vi "cargoLoop.vi"() -> ()   [LabVIEW 2018]
uses:
  <vilib>/Platform/TimedLoop/XDataNode/timing_clust.ctl
  <vilib>/Platform/TimedLoop/XDataNode/nitl_modes.ctl
  <vilib>/Platform/TimedLoop/XDataNode/wakeup.ctl
  <vilib>/Rock Robotics/WPI/Solenoid/WPI_SolenoidValue.ctl
  cargoNotifier.ctl
  cargoEnum.ctl
  <userlib>/836-Library/System/TDMS_V2/Support/TDMS_DevRef.ctl
  <userlib>/836-Library/System/TDMS_V2/Support/Logging_Settings.ctl
  <userlib>/836-Library/System/TDMS_V2/Support/Group_FIFO_Config.ctl
  <userlib>/836-Library/System/TDMS_V2/Support/Channel_FIFO_Config.ctl
  <vilib>/Rock Robotics/WPI/Solenoid/WPI_SolenoidSetEnum.vi
  <vilib>/platform/TimedLoop/XDataNode/XDataNode.xnode
  <vilib>/Platform/TimedLoop/XDataNode/XDNodeRunTimeDep.lvlib
panel:
  in  "Cargo_Shoot_Time Left":dbl=0.16
  in  "Shoot Time Low Rocket":dbl=1.0
  in  "Cargo_Shoot_Time Right":dbl=0.04
  in  "Rocket_High_Shoot_Time":dbl=1.0
  in  "Reset":bool
  out "Data":cluster{i16, i16}(graph)={1, 0}
  out "Right_Out":bool
  out "Left_Out":bool
  out "Shoot_Right?":bool
  out "Shoot_Left?":bool
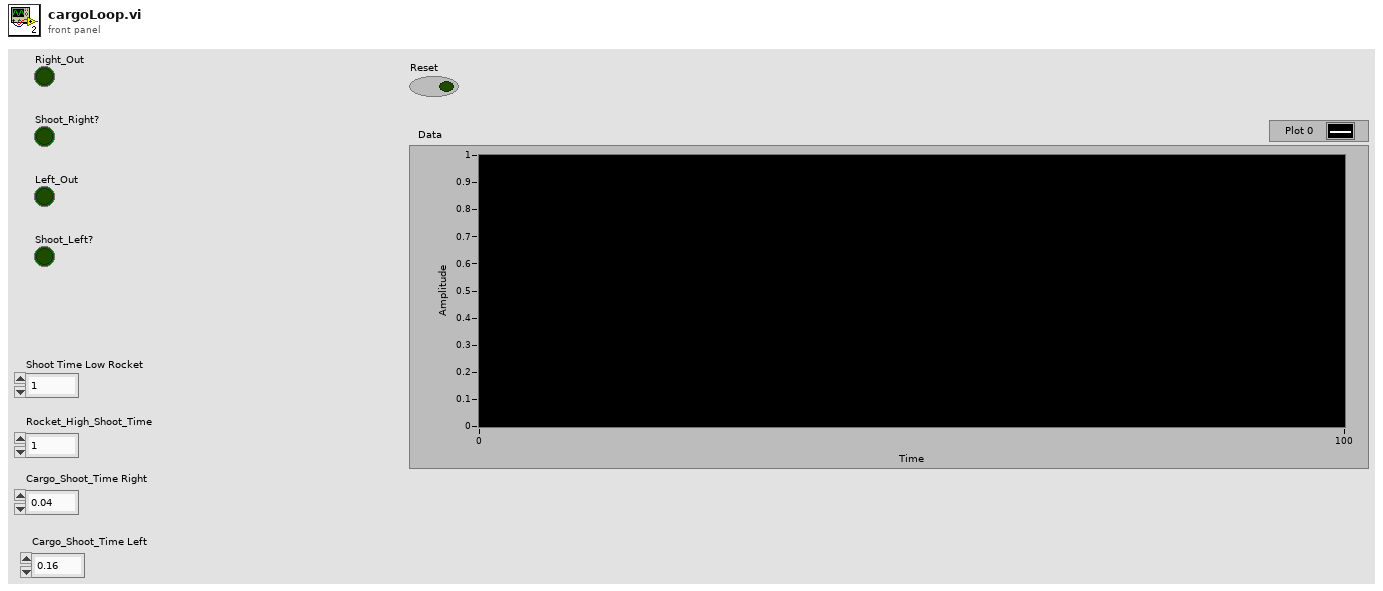
[diagram p1: front panel]
types:
  T1 = typedef "WPI_SolenoidDevRef.ctl" = cluster{"DevStatus":errorcluster, "Pneumatics Control Module":u8, "Forward Solenoid Channel":T2, "Reverse Solenoid Channel":T2}
  T2 = typedef "WPI_SolenoidChannel.ctl" = enum8{"Solenoid 0", "Solenoid 1", "Solenoid 2", "Solenoid 3", "Solenoid 4", "Solenoid 5", "Solenoid 6", "Solenoid 7", "Invalid"}
  T3 = typedef "XDNodeRunTimeDep.lvlib/timing_clust.ctl" = cluster{"Expected End [f-1]":u64, "Actual End [f-1]":u64, "Finished Late? [f-1]":bool, "Expected End [i-1]":u64, "Actual End [i-1]":u64, "Finished Late? [i-1]":bool, "Expected Start [i]":u64, "Actual Start [i]":u64, "Expected Start [f]":u64, "Actual Start [f]":u64, "Source Name":string, "Structure Name":string, "Period":i64, "Deadline":i64, "Offset":i64, "Start":i64, "Priority":i32, "Timeout":i32, "Mode":T4, "Wakeup Reason":T5, "Error":errorcluster, "Source Type":string, "Secondary Source Type":string, "Global End Time":u64, "Global Start Time":u64, "Frame Duration":u64, "Iteration Duration":u64, "Assigned CPU":i32, "I/O Scan Engine Mode":u32}
  T4 = typedef "XDNodeRunTimeDep.lvlib/nitl_modes.ctl" = enum32{"No Change", "Process missed periods, maintain original phase", "Discard missed periods, maintain original phase", "Process missed periods, ignore original phase", "Discard missed periods, ignore original phase"}
  T5 = typedef "XDNodeRunTimeDep.lvlib/wakeup.ctl" = enum32{"Normal", "Aborted", "Asynchronous wakeup", "Timing source error", "Timed loop error", "Timeout"}
  T6 = typedef "WPI_SolenoidValue.ctl" = enum16{"Off", "On", "Forward", "Reverse"}
  T7 = typedef "cargoNotifier.ctl" = cluster{"Cargo State":T8, "Rocket?":bool, "Shoot":bool}
  T8 = typedef "cargoEnum.ctl" = enum16{"do nothing", "rocket right", "rocket left", "cargo ship left", "cargo ship right"}
  T9 = typedef "TDMS_DevRef.ctl" = cluster{"Name":string, "File Ref":refnum<k34>, "Start Time":timestamp, "Logging Settings":T10, "Group FIFO Config":T11[], "Data To Write":refnum<data-value>, "semaphore":T13, "Ref Time Reset":refnum<k4>}
  T10 = typedef "Logging_Settings.ctl" = cluster{"Data Grab Period":dbl, "File Write Period":dbl, "Max Stored Size":dbl, "Burst Size":dbl}
  T11 = typedef "Group_FIFO_Config.ctl" = cluster{"Group":string, "Channels":T12[], "Channel Names":string[]}
  T12 = typedef "Channel_FIFO_Config.ctl" = cluster{"Channel":string, "FIFO":refnum<k33>}
  T13 = typedef "Semaphore RefNum" = refnum<k1>
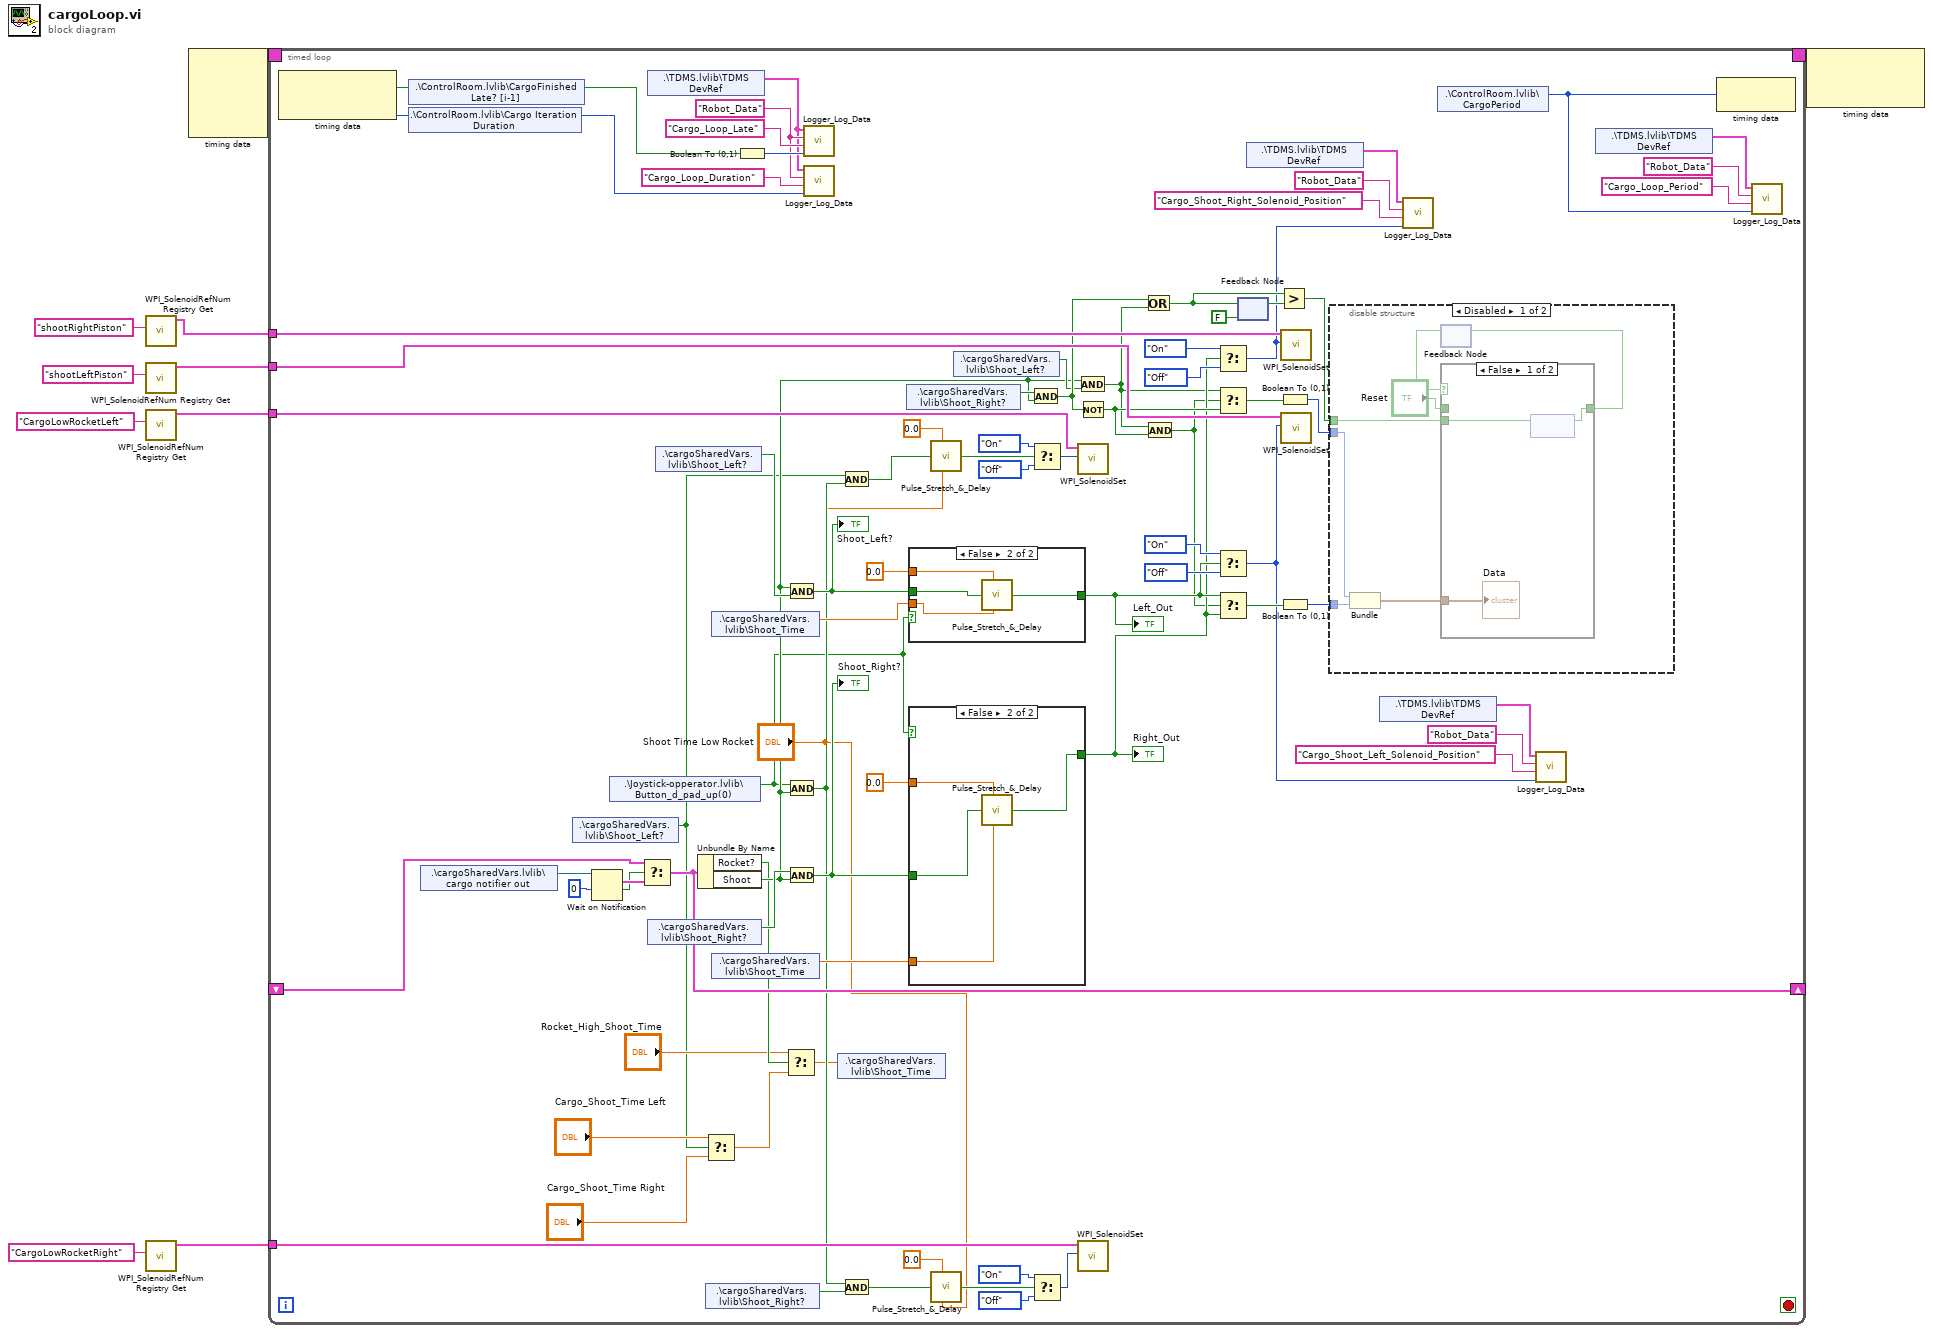
[diagram p0: block diagram]
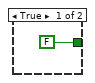
[diagram p2: hidden frame]
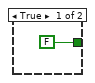
[diagram p3: hidden frame]
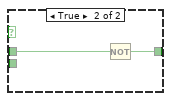
[diagram p4: hidden frame]
diagram:
  n1 = call <vilib>:"WPI_SolenoidRefNum Registry Get.vi"("refnum name"="shootRightPiston") -> ("SolenoidDevRef"=w8:T1)  [unwired: 9 in, 1 out]
  n2 = call <vilib>:"WPI_SolenoidRefNum Registry Get.vi"("refnum name"="shootLeftPiston") -> ("SolenoidDevRef"=w7:T1)  [unwired: 9 in, 1 out]
  n3 = call <vilib>:"WPI_SolenoidRefNum Registry Get.vi"("refnum name"="CargoLowRocketLeft") -> ("SolenoidDevRef"=w2:T1)  [unwired: 9 in, 1 out]
  n4 = call <vilib>:"WPI_SolenoidRefNum Registry Get.vi"("refnum name"="CargoLowRocketRight") -> ("SolenoidDevRef"=w1:T1)  [unwired: 9 in, 1 out]
  n5 = node-c288() -> (w10:T3)  [unwired: 4 in]
  n6 = timed-loop {
    timing: w10 -> [_]
    timing-out: [_] -> w9
    tunnel: w8 -> [w90]
    tunnel: w7 -> [w89]
    shift-right: [w58] -> _
    shift-left: _ -> [w60]
    tunnel: w2 -> [w55]
    tunnel: w1 -> [w54]
    stop <- _ stop-if-true
    w22 = "Robot_Data" ("Group")
    n7 = node-c288() -> (w20:bool, w19:i64)  [unwired: 1 in]
    n8 = shared-variable ".\\ControlRoom.lvlib\\CargoFinished Late? [i-1]"(w20) -> ()  [unwired: 1 in, 1 out]
    n9 = shared-variable ".\\ControlRoom.lvlib\\Cargo Iteration Duration"(w19) -> ()  [unwired: 1 in, 1 out]
    n10 = shared-variable ".\\cargoSharedVars.lvlib\\cargo notifier out"() -> (w62:refnum<notifier>)  [unwired: 1 in, 1 out]
    n11 = shared-variable ".\\cargoSharedVars.lvlib\\Shoot_Left?"() -> (w31:bool)  [unwired: 1 in, 1 out]
    n12 = Wait on Notification(notifier=w62, timeout in ms (-1)=0) -> (notification=w61:T7, timed out?=w59:bool)  [unwired: 2 in, 2 out]
    n13 = shared-variable ".\\Joystick-opperator.lvlib\\Button_d_pad_up(0)"() -> (w35:bool)  [unwired: 1 in, 1 out]
    n14 = Select(t=w60, s=w59, f=w61) -> (s? t:f=w58:T7)
    n15 = shared-variable ".\\TDMS.lvlib\\TDMS DevRef"() -> (w21:T9)  [unwired: 1 in, 1 out]
    n16 = shared-variable ".\\cargoSharedVars.lvlib\\Shoot_Right?"() -> (w91:bool)  [unwired: 1 in, 1 out]
    n17 = shared-variable ".\\cargoSharedVars.lvlib\\Shoot_Left?"() -> (w56:bool)  [unwired: 1 in, 1 out]
    n18 = Unbundle By Name(w58) -> ("Rocket?"=w39:bool, "Shoot"=w40:bool)
    n19 = Select(t="Cargo_Shoot_Time Left", s=w31, f="Cargo_Shoot_Time Right") -> (s? t:f=w34:dbl)
    n20 = shared-variable ".\\cargoSharedVars.lvlib\\Shoot_Right?"() -> (w42:bool)  [unwired: 1 in, 1 out]
    n21 = shared-variable ".\\cargoSharedVars.lvlib\\Shoot_Time"() -> (w80:dbl)  [unwired: 1 in, 1 out]
    n22 = shared-variable ".\\cargoSharedVars.lvlib\\Shoot_Time"() -> (w79:dbl)  [unwired: 1 in, 1 out]
    n23 = Boolean To (0,1)(Boolean=w20) -> (0, 1=w24:i16)
    n24 = Select(t="Rocket_High_Shoot_Time", s=w39, f=w34) -> (s? t:f=w37:dbl)
    n25 = And(x=w40, y=w56) -> (x .and. y?=w64:bool)
    "Shoot_Left?" <- w64
    n26 = And(x=w35, y=w40) -> (x .and. y?=w41:bool)
    n27 = And(x=w91, y=w40) -> (x .and. y?=w66:bool)
    "Shoot_Right?" <- w66
    n28 = call <userlib>:"Logger_Log_Data.vi"("Data"=w24, "Channel"="Cargo_Loop_Late", "Group"=w22, "TDMS DevRef"=w21) -> ()  [unwired: 7 in, 1 out]
    n29 = call <userlib>:"Logger_Log_Data.vi"("Data"=w19, "Channel"="Cargo_Loop_Duration", "Group"=w22, "TDMS DevRef"=w21) -> ()  [unwired: 7 in, 1 out]
    n30 = shared-variable ".\\cargoSharedVars.lvlib\\Shoot_Time"(w37) -> ()  [unwired: 1 in, 1 out]
    n31 = And(x=w31, y=w41) -> (x .and. y?=w44:bool)
    n32 = And(x=w41, y=w42) -> (x .and. y?=w45:bool)
    n33 = shared-variable ".\\cargoSharedVars.lvlib\\Shoot_Right?"() -> (w69:bool)  [unwired: 1 in, 1 out]
    n34 = case shown="False" w35 {
      tunnel: 0.0 ("Delay (sec)") -> [_ w96]
      tunnel: w80 -> [_ w95]
      tunnel: [FALSE ("Out") w94] -> w75
      tunnel: w64 -> [_ w93]
      frame True {
      }
      frame False {
        n35 = call <userlib>:"Pulse_Stretch_&_Delay.vi"("Delay (sec)"=w96, "In"=w93, "Width (sec)"=w95) -> ("Out"=w94:bool)  [unwired: 2 in]
      }
    }
    "Left_Out" <- w75
    n36 = case shown="False" w35 {
      tunnel: 0.0 ("Delay (sec)") -> [_ w101]
      tunnel: w79 -> [_ w100]
      tunnel: [FALSE ("Out") w99] -> w74
      tunnel: w66 -> [_ w98]
      frame True {
      }
      frame False {
        n37 = call <userlib>:"Pulse_Stretch_&_Delay.vi"("Delay (sec)"=w101, "In"=w98, "Width (sec)"=w100) -> ("Out"=w99:bool)  [unwired: 2 in]
      }
    }
    "Right_Out" <- w74
    n38 = call <userlib>:"Pulse_Stretch_&_Delay.vi"("Delay (sec)"=0.0, "In"=w44, "Width (sec)"="Shoot Time Low Rocket") -> ("Out"=w43:bool)  [unwired: 2 in]
    n39 = call <userlib>:"Pulse_Stretch_&_Delay.vi"("Delay (sec)"=0.0, "In"=w45, "Width (sec)"="Shoot Time Low Rocket") -> ("Out"=w46:bool)  [unwired: 2 in]
    n40 = shared-variable ".\\cargoSharedVars.lvlib\\Shoot_Left?"() -> (w57:bool)  [unwired: 1 in, 1 out]
    n41 = And(x=w69, y=w40) -> (x .and. y?=w67:bool)
    n42 = Select(t=WPI_SolenoidValue."On" ("Value"), s=w43, f=WPI_SolenoidValue."Off" ("Value")) -> (s? t:f=w48:T6)
    n43 = Select(t=WPI_SolenoidValue."On" ("Value"), s=w46, f=WPI_SolenoidValue."Off" ("Value")) -> (s? t:f=w51:T6)
    n44 = And(x=w40, y=w57) -> (x .and. y?=w65:bool)
    n45 = Not(x=w67) -> (.not. x?=w78:bool)
    n46 = call-poly <vilib>:"WPI_SolenoidSet.vi"("Value"=w48, "SolenoidDevRef"=w55) -> ()  [unwired: 8 in, 2 out]
    n47 = call-poly <vilib>:"WPI_SolenoidSet.vi"("Value"=w51, "SolenoidDevRef"=w54) -> ()  [unwired: 8 in, 2 out]
    n48 = Or(x=w67, y=w65) -> (x .or. y?=w71:bool)
    n49 = And(x=w65, y=w78) -> (x .and. y?=w73:bool)
    n50 = Select(t=WPI_SolenoidValue."On" ("Value"), s=w74, f=WPI_SolenoidValue."Off" ("Value")) -> (s? t:f=w15:T6)
    n51 = Select(t=w65, s=w73, f=w78) -> (s? t:f=w82:bool)
    n52 = Select(t=WPI_SolenoidValue."On" ("Value"), s=w75, f=WPI_SolenoidValue."Off" ("Value")) -> (s? t:f=w11:T6)
    n53 = Select(t=w75, s=w73, f=w74) -> (s? t:f=w81:bool)
    n54 = feedback-in #1(w71) -> ()
    n55 = feedback #1(FALSE) -> (w72:bool)
    n56 = shared-variable ".\\TDMS.lvlib\\TDMS DevRef"() -> (w17:T9)  [unwired: 1 in, 1 out]
    n57 = Greater?(x=w71, y=w72) -> (0:w68:bool)
    n58 = Boolean To (0,1)(Boolean=w82) -> (0, 1=w77:i16)
    n59 = Boolean To (0,1)(Boolean=w81) -> (0, 1=w76:i16)
    n60 = call-poly <vilib>:"WPI_SolenoidSet.vi"("Value"=w15, "SolenoidDevRef"=w90) -> ()  [unwired: 8 in, 2 out]
    n61 = call-poly <vilib>:"WPI_SolenoidSet.vi"("Value"=w11, "SolenoidDevRef"=w89) -> ()  [unwired: 8 in, 2 out]
    n62 = disable-structure shown="Disabled" {
      disable-tunnel: w77 -> [w107 _]
      disable-tunnel: w76 -> [w106 _]
      disable-tunnel: w68 -> [w105 _]
      frame Disabled {
        n63 = Bundle(w107, w106) -> (w108:cluster{i16, i16})  [unwired: 1 in]
        n64 = feedback #2() -> (w103:bool)  [unwired: 1 in]
        n65 = case shown="False" w103 {
          tunnel: w108 -> [w111 _]
          tunnel: w105 -> [w110 _]
          tunnel: [w109 w113] -> w104
          tunnel: "Reset" -> [_ w112]
          frame False {
            n66 = feedback #3() -> (w109:bool)  [unwired: 1 in]
            n67 = feedback-in #3(w110) -> ()
            "Data" <- w111
          }
          frame True {
            n68 = Not(x=w112) -> (.not. x?=w113:bool)
          }
        }
        n69 = feedback-in #2(w104) -> ()
      }
      frame Enabled {
      }
    }
    n70 = shared-variable ".\\TDMS.lvlib\\TDMS DevRef"() -> (w13:T9)  [unwired: 1 in, 1 out]
    n71 = call <userlib>:"Logger_Log_Data.vi"("Data"=w15, "Channel"="Cargo_Shoot_Right_Solenoid_Position", "Group"="Robot_Data", "TDMS DevRef"=w17) -> ()  [unwired: 7 in, 1 out]
    n72 = shared-variable ".\\ControlRoom.lvlib\\CargoPeriod"() -> (w26:i64)  [unwired: 1 in, 1 out]
    n73 = call <userlib>:"Logger_Log_Data.vi"("Data"=w11, "Channel"="Cargo_Shoot_Left_Solenoid_Position", "Group"="Robot_Data", "TDMS DevRef"=w13) -> ()  [unwired: 7 in, 1 out]
    n74 = shared-variable ".\\TDMS.lvlib\\TDMS DevRef"() -> (w28:T9)  [unwired: 1 in, 1 out]
    n75 = node-c288(w26) -> ()  [unwired: 1 out]
    n76 = call <userlib>:"Logger_Log_Data.vi"("Data"=w26, "Channel"="Cargo_Loop_Period", "Group"="Robot_Data", "TDMS DevRef"=w28) -> ()  [unwired: 7 in, 1 out]
  }
  n77 = node-c288(w9) -> ()  [unwired: 2 out]
